vi "Main.vi"   [LabVIEW 2019]
uses:
  03_Home/controller/pannelState.ctl
  globalValue.vi
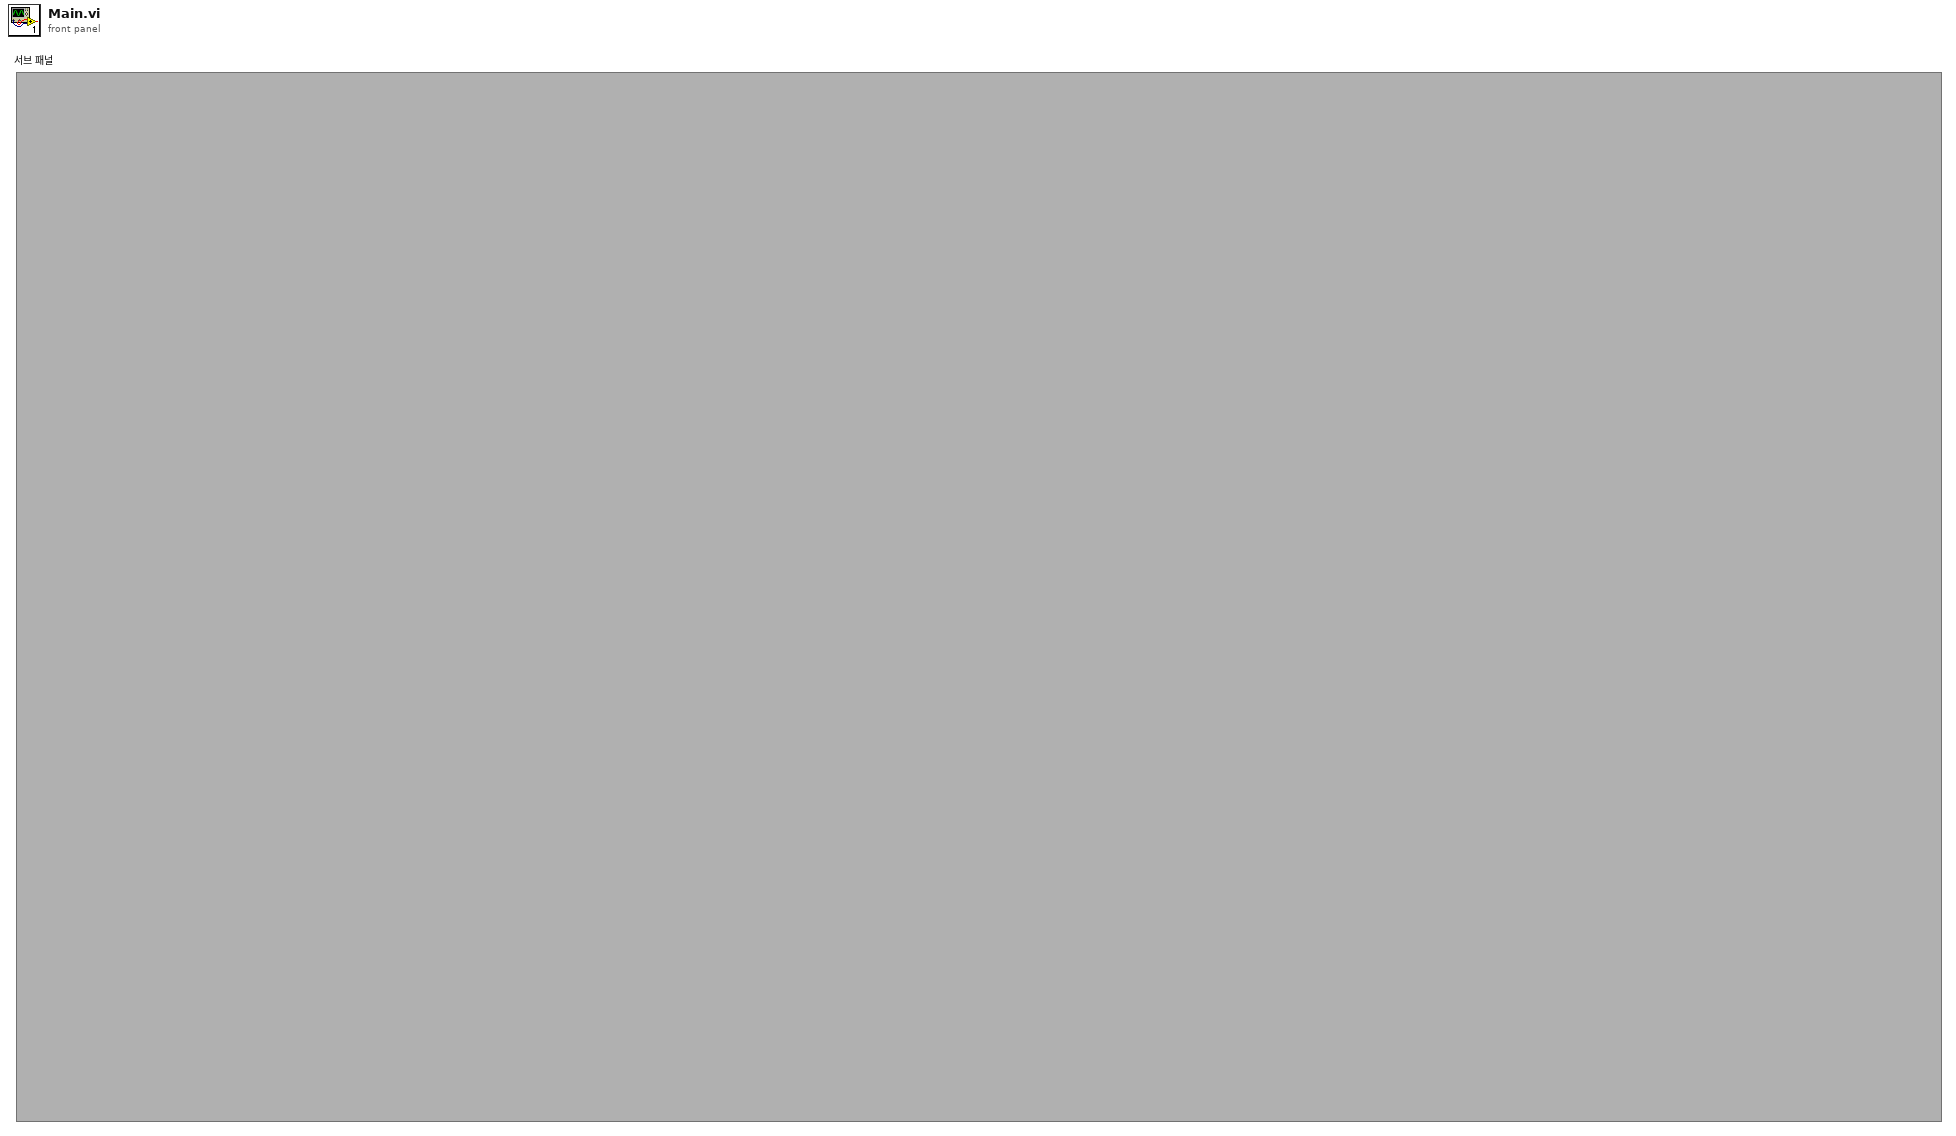
[diagram p1: front panel]
types:
  T1 = typedef "pannelState.ctl" = enum16{"Init", "LogIn", "SignUpView", "Home", "Management_patientList", "Management_patientTrashtList", "Management_patientCreate", "Management_patientUpdate", "Management_patientTraining", "Management_patientTrainingDetail", "H-MEDI PatientList", "H-MEDI HardwareCtl", "Adjust", "FineTuning", "UserList", "UserDetail", "Exit"}
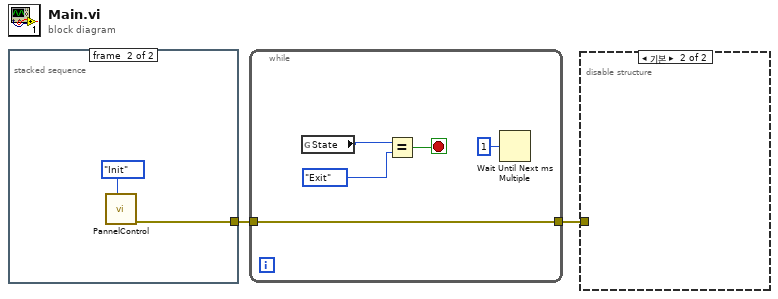
[diagram p0: block diagram]
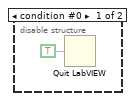
[diagram p2: hidden frame]
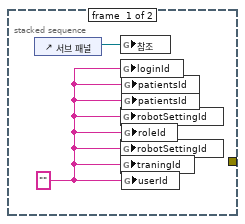
[diagram p3: hidden frame]
diagram:
  n1 = stacked-sequence {
    tunnel: [_ w5] -> w2
    frame #0 {
      w3 = ""
      n2 = control-ref of="서브 패널"() -> (w4:refnum<vi>)
      n3 = global write "globalValue.vi" "참조"(w4) -> ()
      n4 = global write "globalValue.vi" "loginId"(w3) -> ()
      n5 = global write "globalValue.vi" "robotSettingId"(w3) -> ()
      n6 = global write "globalValue.vi" "robotSettingId"(w3) -> ()
      n7 = global write "globalValue.vi" "traningId"(w3) -> ()
      n8 = global write "globalValue.vi" "patientsId"(w3) -> ()
      n9 = global write "globalValue.vi" "patientsId"(w3) -> ()
      n10 = global write "globalValue.vi" "roleId"(w3) -> ()
      n11 = global write "globalValue.vi" "userId"(w3) -> ()
    }
    frame #1 {
      n12 = call "PannelControl.vi"("State"=pannelState."Init") -> ("error out"=w5:errorcluster)  [unwired: 10 in]
    }
  }
  n13 = while {
    tunnel: w2 -> [w7]
    tunnel: [w7] -> w1
    stop <- w9 stop-if-true
    n14 = global read "globalValue.vi" "State"() -> (w11:T1)
    n15 = Equal?(x=w11, y=pannelState."Exit" ("State")) -> (x = y?=w9:bool)
    n16 = Wait Until Next ms Multiple(millisecond multiple=u32 1 ("ms 배수")) -> ()  [unwired: 1 out]
  }
  n17 = disable-structure shown="기본" {
    disable-tunnel: w1 -> [_ _]
    frame condition #0 {
      n18 = Quit LabVIEW(quit? (T)=TRUE ("종료? (참)")) -> ()
    }
    frame condition #1 (active) {
    }
  }
